vi "SaveResultFile.vi"(6 "Overwrite":bool, 8 "error in (no error)":errorcluster, 10 "FolderPath":path, 11 "CAlexData2 in":refnum<class "CAlex2_Data.lvclass">) -> (0 "error out":errorcluster, 1 "FileName":string, 2 "FilePath":path, 3 "CAlexData2 out":refnum<class "CAlex2_Data.lvclass">)   [LabVIEW 2015, in "CAlex2_Data.lvclass"]
uses:
  CAlex2_Data.lvclass
  <vilib>/Utility/file.llb/Write Delimited Spreadsheet (DBL).vi
  <vilib>/GoldZinc Software/auzn custom VIs/CustomVI.lvlib
panel:
  in  "Dilate Length":i32=500
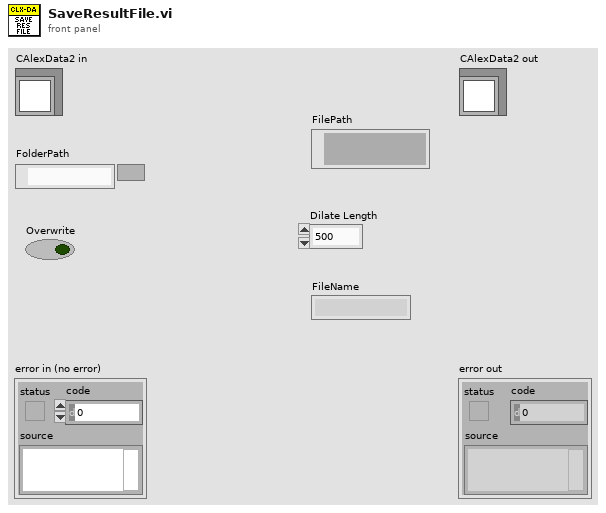
[diagram p1: front panel]
types:
  T1 = enum16{"open", "replace", "create", "open or create", "replace or create", "replace or create with confirmation"}
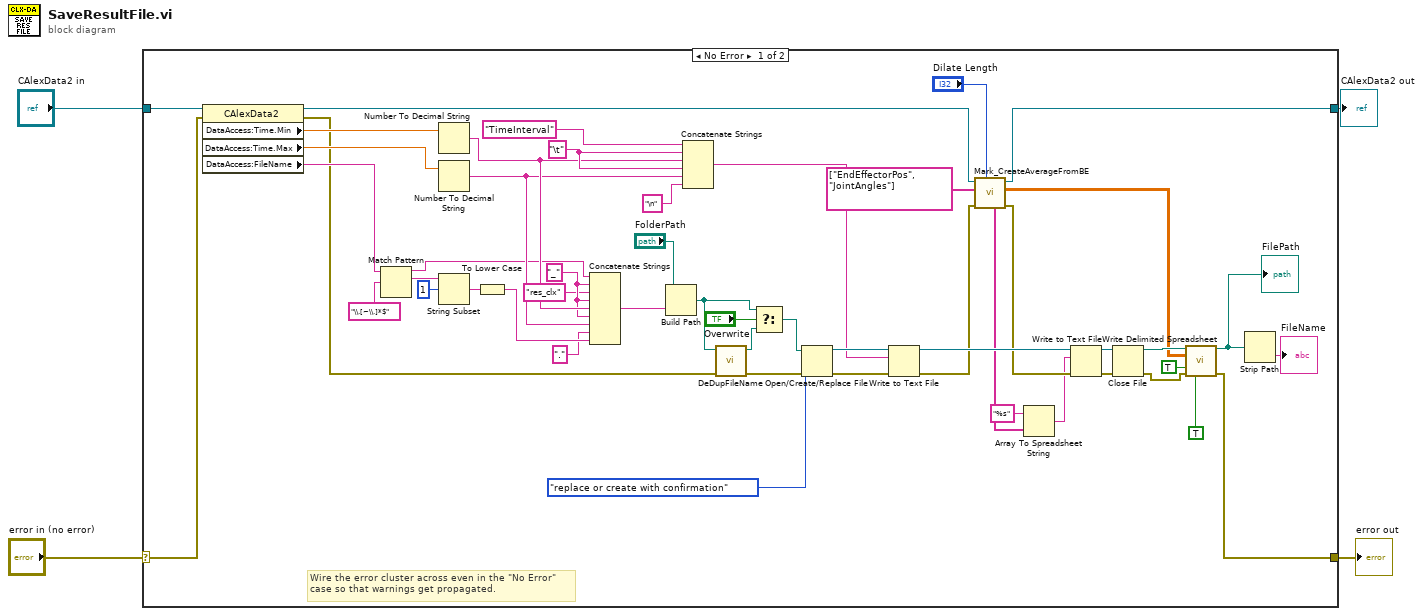
[diagram p0: block diagram]
diagram:
  n1 = case shown="No Error" "error in (no error)" {
    selector: "error in (no error)" -> [w53 w57]
    tunnel: [w11 w57] -> w3
    tunnel: [w44 w56] -> w1
    tunnel: "CAlexData2 in" -> [w54 w56]
    frame No Error {
      w18 = "_" ("string")
      w49 = "\t" ("string")
      # "Wire the error cluster across even in the \"No Error\"\ncase so that warnings get propagated."
      n2 = property class="CAlexData2"(reference=w54, error in=w53) -> (reference out=w45:refnum<class "CAlex2_Data.lvclass">, error out=w15:errorcluster, "DataAccess:Time.Min"=w52:dbl, "DataAccess:Time.Max"=w51:dbl, "DataAccess:FileName"=w26:string)
      n3 = Match Pattern(string=w26, regular expression="\\.[~\\.]*$") -> (before substring=w19:string, match substring=w27:string)  [unwired: 3 out]
      n4 = Number To Decimal String(number=w52) -> (decimal integer string=w48:string)  [unwired: 1 in]
      n5 = Number To Decimal String(number=w51) -> (decimal integer string=w47:string)  [unwired: 1 in]
      n6 = String Subset(string=w27, offset (0)=1) -> (substring=w28:string)  [unwired: 1 out]
      n7 = To Lower Case(string=w28) -> (all lower case string=w25:string)
      n8 = Concatenate Strings(w19, w18, "res_clx" ("string"), w18, w48, w18, w47, "." ("string"), w25) -> (w46:string)
      n9 = Build Path(base path="FolderPath", name or relative path=w46) -> (appended path=w8:path)
      n10 = Concatenate Strings("TimeInterval", w49, w48, w49, w47, "\n" ("string")) -> (w40:string)
      n11 = call <vilib>:"DeDupFileName.vi"("error in (no error)"=w15, "Path"=w8) -> ("error out"=w43:errorcluster, "Out Path"=w10:path)  [unwired: 7 in, 1 out]
      n12 = Select(t=w8, s="Overwrite", f=w10) -> (s? t:f=w9:path)
      n13 = Open/Create/Replace File(file path (use dialog)=w9, error in=w43, operation (0:open)=T1."replace or create with confirmation") -> (refnum out=w41:refnum<file>, error out=w42:errorcluster)  [unwired: 3 in, 1 out]
      n14 = Write to Text File(file (use dialog)=w41, text=w40, error in=w42) -> (refnum out=w36:refnum<file>, error out=w32:errorcluster)  [unwired: 1 in, 1 out]
      n15 = call-dynamic "Mark_CreateAverageFromBE.vi"("Dilate Length"="Dilate Length", "error in (no error)"=w32, "Variables"=string[] ["EndEffectorPos", "JointAngles"], "ExpData in"=w45) -> ("error out"=w31:errorcluster, "Mean"=w37:dbl[][], "ExpData out"=w44:refnum<class "CAlex2_Data.lvclass">, "ColHeaders"=w23:string[])  [unwired: 3 in, 1 out]
      n16 = Array To Spreadsheet String(array=w23, 3:"%s" ("format string")) -> (spreadsheet string=w22:string)  [unwired: 1 in]
      n17 = Write to Text File(file (use dialog)=w36, text=w22, error in=w31) -> (refnum out=w35:refnum<file>, error out=w34:errorcluster)  [unwired: 1 in, 1 out]
      n18 = Close File(refnum=w35, error in=w34) -> (path=w38:path, error out=w12:errorcluster)
      n19 = call-poly <vilib>:"Write Delimited Spreadsheet.vi"("file path (dialog if empty)"=w38, "2D data"=w37, "append to file? (F)"=TRUE ("append to file? (new file:F)"), "error in (no error)"=w12, "transpose? (F)"=TRUE ("transpose? (no:F)")) -> ("new file path (Not A Path if cancelled)"=w6:path, "error out"=w11:errorcluster)  [unwired: 9 in]
      "FilePath" <- w6
      n20 = Strip Path(path=w6) -> (name=→"FileName":string)  [unwired: 1 out]
    }
    frame Error {
    }
  }
  "error out" <- w3
  "CAlexData2 out" <- w1
